vi "Get Tag by Index.vi"(8 "error in (no error)":errorcluster, 9 "Index":i32, 10 "Parent Tag":string, 11 "Tag Tree Helper In":refnum<class "Tag Tree Helper.lvclass">) -> (0 "error out":errorcluster, 2 "Tag":string, 3 "Tag Tree Helper Out":refnum<class "Tag Tree Helper.lvclass">)   [LabVIEW 2020, in "Process Generation.lvlib" / "Tag Tree Helper.lvclass"]
uses:
  Tag Tree Helper.lvclass
  Tag Tree Helper.lvclass/Tag Tree Helper.ctl
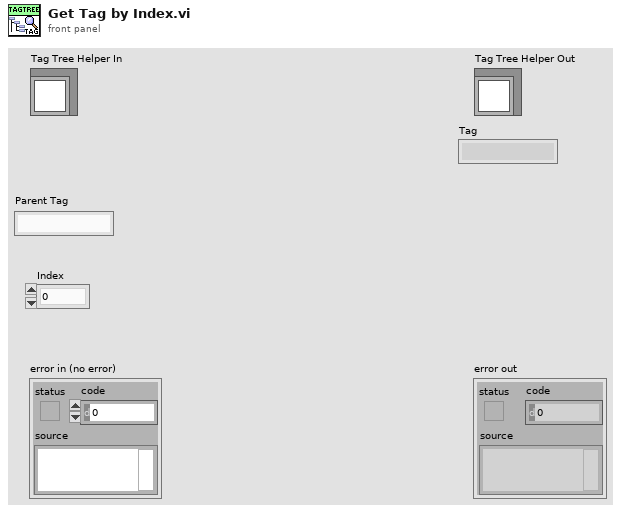
[diagram p1: front panel]
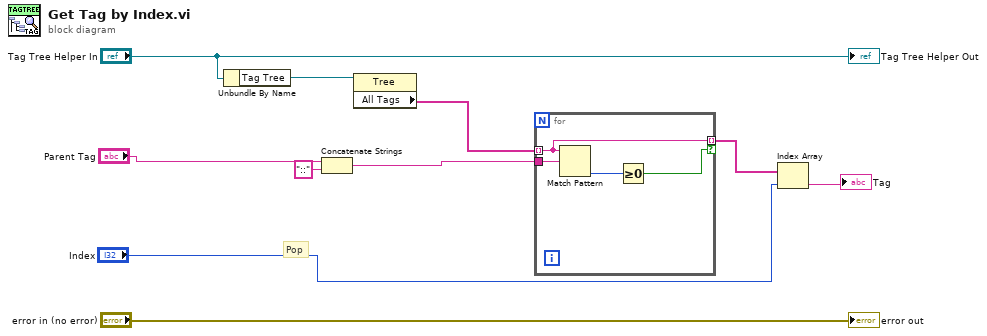
[diagram p0: block diagram]
diagram:
  # "Pop"
  n1 = Unbundle By Name("Tag Tree Helper In") -> ("Tag Tree"=w8:refnum<vi>)
  n2 = Concatenate Strings("Parent Tag", "::" ("string")) -> (w2:string)
  n3 = property class="Tree"(reference=w8) -> ("All Tags"=w7:string[])  [unwired: 1 in, 2 out]
  n4 = for {
    tunnel: w7 -> [w12] mode=indexing
    tunnel: w2 -> [w14]
    tunnel: [w12] -> w5 mode=indexing if=w11
    n5 = Match Pattern(string=w12, regular expression=w14) -> (offset past match=w13:i32)  [unwired: 1 in, 3 out]
    n6 = Greater Or Equal To 0?(x=w13) -> (x >= 0?=w11:bool)
  }
  n7 = Index Array(array=w5, index="Index") -> (element=→"Tag":string)
  "error out" <- "error in (no error)"
  "Tag Tree Helper Out" <- "Tag Tree Helper In"
